vi "Write data member A.vi"(8 "error in (no error)":errorcluster, 10 "Data member A":dbl, 11 "Sample Class in":refnum<class "Sample Class.lvclass">) -> (0 "error out":errorcluster, 3 "Sample Class out":refnum<class "Sample Class.lvclass">)   [LabVIEW 2023, in "Sample Class.lvclass"]
doc: "Writes a value for Data member A into an instance of Sample class."
uses:
  Sample Class.lvclass
  Sample Class.lvclass/Sample Class.ctl
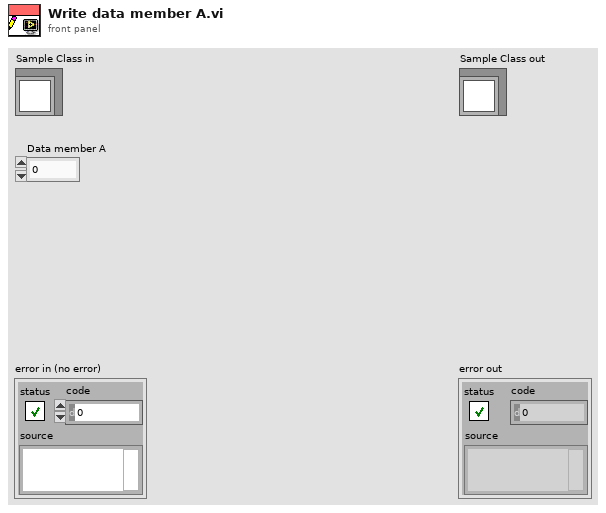
[diagram p1: front panel]
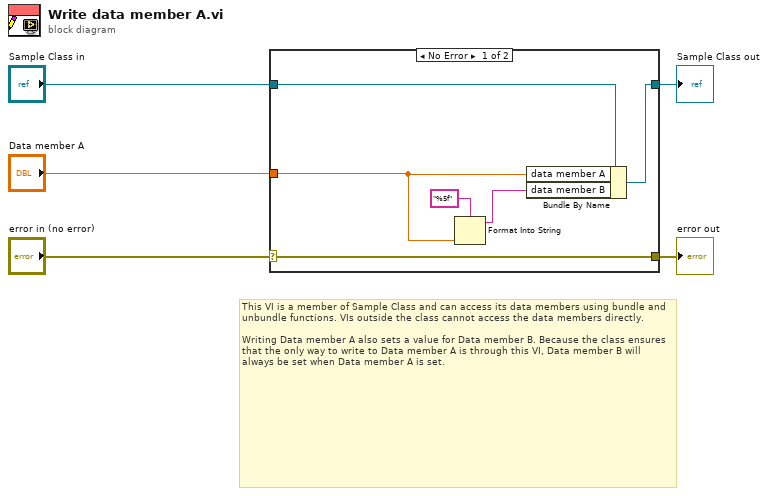
[diagram p0: block diagram]
diagram:
  # "This VI is a member of Sample Class and can access its data members using bundle and unbundle functions. VIs outside the class cannot access the data members directly.\n\nWriting Data member A also sets a value for Data member B. Because the class ensures that the only way to write to Data member A is through this VI, Data member B will always be set when Data member A is set."
  n1 = case shown="No Error" "error in (no error)" {
    selector: "error in (no error)" -> [w11 w12]
    tunnel: [w11 w12] -> w4
    tunnel: [w9 w13] -> w2
    tunnel: "Sample Class in" -> [w10 w13]
    tunnel: "Data member A" -> [w8 _]
    frame No Error {
      n2 = Format Into String(format string="%5f", w8) -> (resulting string=w7:string)  [unwired: 2 in, 1 out]
      n3 = Bundle By Name(cluster=w10, "data member A"=w8, "data member B"=w7) -> (w9:refnum<class "Sample Class.lvclass">)
    }
    frame Error {
    }
  }
  "error out" <- w4
  "Sample Class out" <- w2
